vi "mapTo2DArr.vi"(1 "Map":map{u32, u32}(c390)) -> (0 "2D Array":i32[][](array[numeric]))   [LabVIEW 2019]
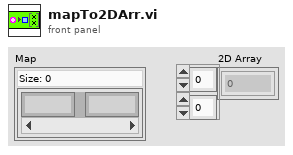
[diagram p1: front panel]
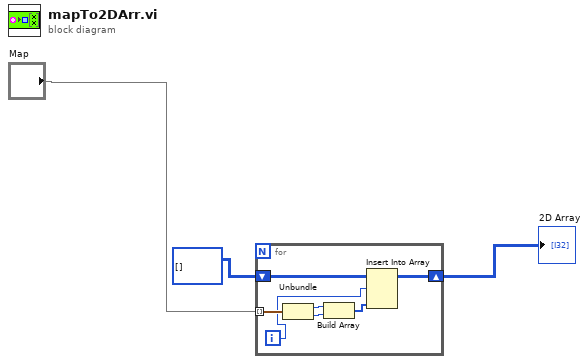
[diagram p0: block diagram]
diagram:
  n1 = for {
    tunnel: "Map" -> [w10] mode=indexing
    shift-right: [w8] -> w3
    shift-left: i32[][] [] -> [w9]
    i -> [w4]
    n2 = Unbundle(w10) -> ("key"=w7:u32, "value"=w6:u32)
    n3 = Build Array(w7, w6) -> (w5:u32[])
    n4 = Insert Into Array(array=w9, index (row)=w4, new element=w5) -> (w8:i32[][])  [unwired: 1 in]
  }
  "2D Array" <- w3
